vi "Current Convert test.vi"() -> ()   [LabVIEW 2013]
panel:
  out "z 2":dbl
  out "y 2":dbl
  out "x 2":dbl
  in  "Z 2":dbl
  in  "Y 2":dbl
  in  "X 2":dbl
  out "z":dbl
  out "y":dbl
  out "x":dbl
  in  "Z":dbl
  in  "Y":dbl
  in  "X":dbl
  in  "Table":T1={"Far Left"={"Object"={"X"=70.0, "Y"=70.0, "Z"=0.0, "A"=0.0}, "Robot"={"X"=635.6667183088158, "Y"=-157.45515965253327, "Z"=-104.0, "A"=-2.2592664468744745}}, "Far Right"={"Object"={"X"=70.0, "Y"=-70.0, "Z"=0.0, "A"=0.0}, "Robot"={"X"=633.6829491032604, "Y"=-298.6066739327545, "Z"=-104.0, "A"=-2.7992504924949793}}, "Near Left"={"Object"={"X"=-70.0, "Y"=70.0, "Z"=0.0, "A"=0.0}, "Robot"={"X"=501.946047013151, "Y"=-154.5017752565065, "Z"=-104.0, "A"=-3.895959042500226}}, "Near Right"={"Object"={"X"=-70.0, "Y"=-70.0, "Z"=0.0, "A"=0.0}, "Robot"={"X"=494.37297853464617, "Y"=-294.48684679684237, "Z"=-104.0, "A"=-3.4395881102375703}}}
  # "Basic Commands are:\n   Convert   - convert offset to joints\n   Current   - current joint and offset\n   Save      - save calibration data\n   Load      - load calibration data\n   Reference - give reference joint position"
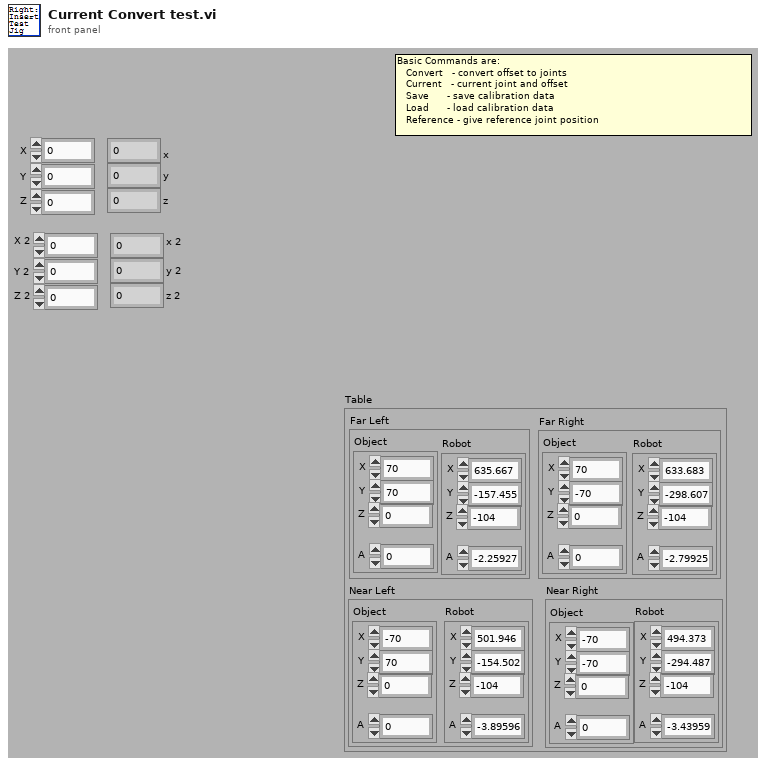
[diagram p1: front panel]
types:
  T1 = cluster{"Far Left":cluster{"Object":cluster{"X":dbl, "Y":dbl, "Z":dbl, "A":dbl}, "Robot":cluster{"X":dbl, "Y":dbl, "Z":dbl, "A":dbl}}, "Far Right":cluster{"Object":cluster{"X":dbl, "Y":dbl, "Z":dbl, "A":dbl}, "Robot":cluster{"X":dbl, "Y":dbl, "Z":dbl, "A":dbl}}, "Near Left":cluster{"Object":cluster{"X":dbl, "Y":dbl, "Z":dbl, "A":dbl}, "Robot":cluster{"X":dbl, "Y":dbl, "Z":dbl, "A":dbl}}, "Near Right":cluster{"Object":cluster{"X":dbl, "Y":dbl, "Z":dbl, "A":dbl}, "Robot":cluster{"X":dbl, "Y":dbl, "Z":dbl, "A":dbl}}}
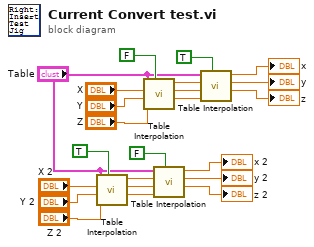
[diagram p0: block diagram]
diagram:
  n1 = call "Table Interpolation.vi"("Invert"=TRUE, "Z"="Z 2", "Y"="Y 2", "X"="X 2", "Table"="Table") -> ("z"=w8:dbl, "y"=w9:dbl, "x"=w10:dbl)  [unwired: 3 in, 1 out]
  n2 = call "Table Interpolation.vi"("Invert"=FALSE, "Z"="Z", "Y"="Y", "X"="X", "Table"="Table") -> ("z"=w19:dbl, "y"=w20:dbl, "x"=w21:dbl)  [unwired: 3 in, 1 out]
  n3 = call "Table Interpolation.vi"("Invert"=FALSE, "Z"=w8, "Y"=w9, "X"=w10, "Table"="Table") -> ("z"=→"z 2":dbl, "y"=→"y 2":dbl, "x"=→"x 2":dbl)  [unwired: 3 in, 1 out]
  n4 = call "Table Interpolation.vi"("Invert"=TRUE, "Z"=w19, "Y"=w20, "X"=w21, "Table"="Table") -> ("z"=→"z":dbl, "y"=→"y":dbl, "x"=→"x":dbl)  [unwired: 3 in, 1 out]
